vi "Error Query.vi"(8 "error in (no error)":errorcluster, 11 "VISA resource name":refnum<visa-resource-name>) -> (0 "error out":errorcluster, 1 "Error Message":string, 2 "Error Code":i32[](array[numeric]), 3 "VISA resource name out":refnum<visa-resource-name>)   [LabVIEW 2013, in "Keithley 2200 Series.lvlib"]
doc: "Queries the instrument for any errors in the instrument's error queue. It will continue to read errors until all errors have been read from the instrument. Any errors will be returned in the Error Out cluster.\n\nNote:\nThis VI is called automatically by most driver VIs so it is not usually necessary to call this in an application."
uses:
  Keithley 2200 Series.lvlib
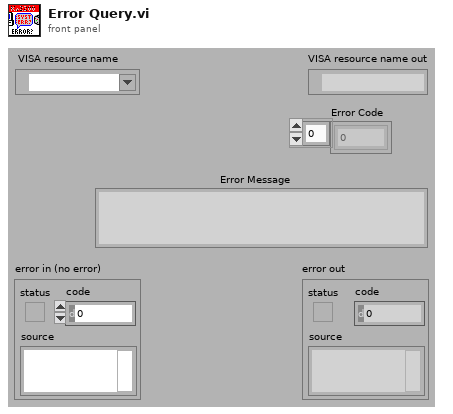
[diagram p1: front panel]
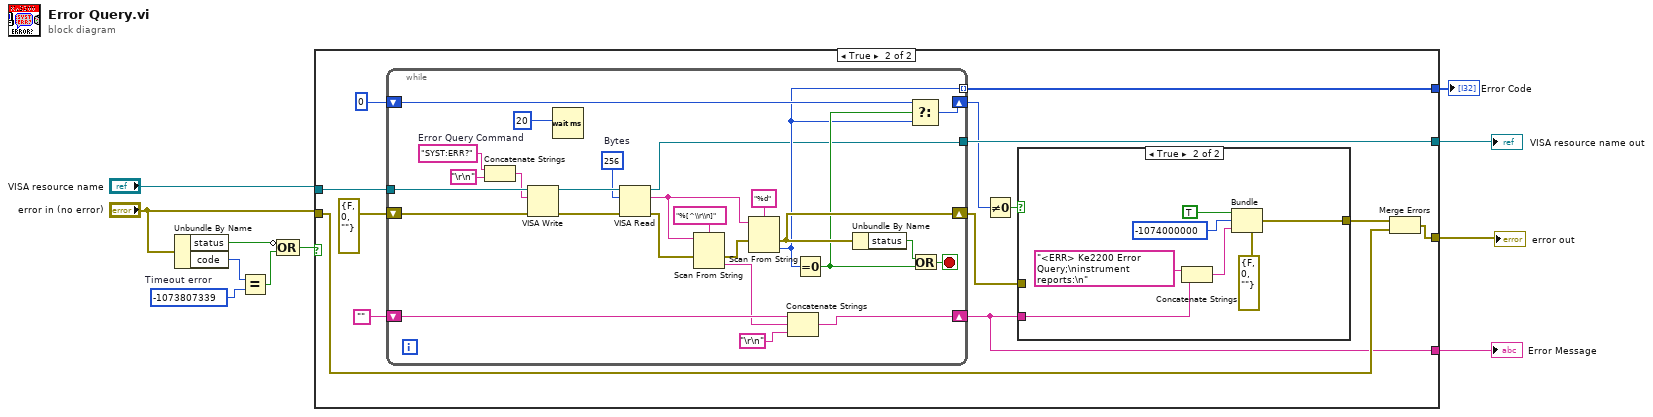
[diagram p0: block diagram]
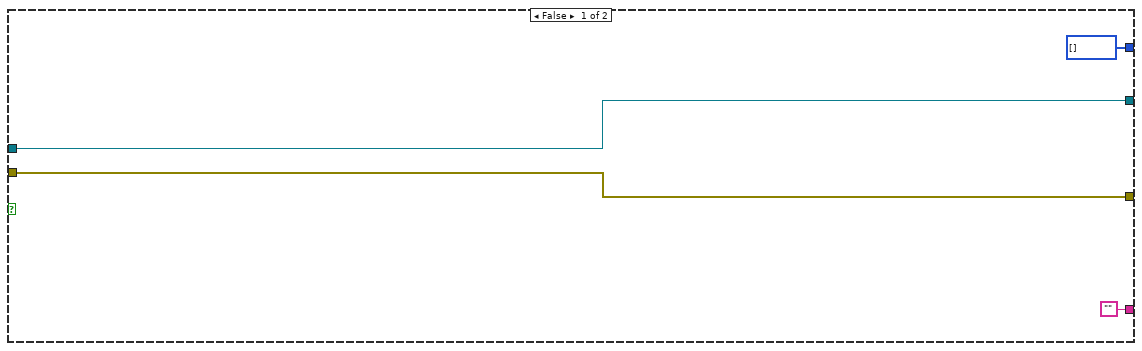
[diagram p2: hidden frame]
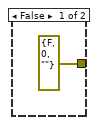
[diagram p3: hidden frame]
diagram:
  w10 = -1073807339  # Timeout error
  n1 = Unbundle By Name("error in (no error)") -> ("status"=w11:bool, "code"=w8:i32)
  n2 = Equal?(x=w8, y=w10) -> (x = y?=w9:bool)
  n3 = Compound Arithmetic op=OR(invert w11, w9) -> (w7:bool)
  n4 = case shown="True" w7 {
    tunnel: [w15 w28] -> w2
    tunnel: "VISA resource name" -> [w15 w27]
    tunnel: "error in (no error)" -> [w14 w21]
    tunnel: [w14 w25] -> w3
    tunnel: ["" ("Empty String Constant") w18] -> w4
    tunnel: [i32[] [] w17] -> w1
    frame False {
    }
    frame True {
      n5 = while {
        tunnel: [w39] -> w17 mode=indexing
        shift-left: errorcluster {"status"=FALSE, "code"=0, "source"=""} ("error in (no error)") -> [w44]
        shift-right: [w43] -> w16
        shift-left: 0 -> [w46]
        shift-right: [w45] -> w19
        shift-left: "" ("Empty String Constant") -> [w50]
        shift-right: [w47] -> w18
        tunnel: w27 -> [w54]
        tunnel: [w37] -> w28
        stop <- w52 stop-if-true
        w36 = u32 256  # Bytes
        w33 = "SYST:ERR?"  # Error Query Command
        n6 = Concatenate Strings(w33, "\r\n" ("End of Line Constant")) -> (w32:string)
        n7 = VISA Write(VISA resource name=w54, write buffer=w32, error in (no error)=w44) -> (VISA resource name out=w38:refnum<visa-resource-name>, error out=w30:errorcluster)  [unwired: 1 out]
        n8 = Wait (ms)(milliseconds to wait=u32 20) -> ()  [unwired: 1 out]
        n9 = VISA Read(VISA resource name=w38, byte count=w36, error in (no error)=w30) -> (VISA resource name out=w37:refnum<visa-resource-name>, read buffer=w34:string, error out=w35:errorcluster)  [unwired: 1 out]
        n10 = Scan From String(format string="%[^\\r\\n]", input string=w34, error in=w35) -> (error out=w42:errorcluster, output 1=w48:string)  [unwired: 1 in, 3 out]
        n11 = Scan From String(format string="%d", input string=w34, error in=w42) -> (error out=w43:errorcluster, output 1=w39:i32)  [unwired: 1 in, 3 out]
        n12 = Concatenate Strings(w50, w48, "\r\n" ("End of Line Constant")) -> (w47:string)
        n13 = Equal To 0?(x=w39) -> (x = 0?=w40:bool)
        n14 = Unbundle By Name(w43) -> ("status"=w41:bool)
        n15 = Select(t=w46, s=w40, f=w39) -> (s? t:f=w45:i32)
        n16 = Or(x=w41, y=w40) -> (x .or. y?=w52:bool)
      }
      n17 = Not Equal To 0?(x=w19) -> (x != 0?=w23:bool)
      n18 = case shown="True" w23 {
        tunnel: w18 -> [_ w58]
        tunnel: [errorcluster {"status"=FALSE, "code"=0, "source"=""} ("error out") w57] -> w22
        tunnel: w16 -> [_ _]
        frame False {
        }
        frame True {
          n19 = Concatenate Strings("<ERR> Ke2200 Error Query;\ninstrument reports:\n" ("Source"), w58) -> (w59:string)
          n20 = Bundle(cluster=errorcluster {"status"=FALSE, "code"=0, "source"=""} ("error out"), "status"=TRUE ("Status"), "code"=-1074000000 ("Code"), "source"=w59) -> (w57:errorcluster)
        }
      }
      n21 = Merge Errors(w22, w21) -> (w25:errorcluster)
    }
  }
  "VISA resource name out" <- w2
  "error out" <- w3
  "Error Message" <- w4
  "Error Code" <- w1
